vi "Day 3-1.vi"() -> ()   [LabVIEW 2019, in "Day 3.lvlib"]
uses:
  <vilib>/Utility/error.llb/Error Cluster From Error Code.vi
  <vilib>/ErrorRing/Error Ring.xnode
  Day 3.lvlib
panel:
  out "Array 3":bool[][](array[boolean])
  out "x*y":u32
  out "epsilon num":u32
  out "gama num":u32
  out "epsilon":bool[](array[boolean])
  out "gama":bool[](array[boolean])
  out "Array 2":bool[][](array[boolean])
  out "error IO":errorcluster
  out "Array":string[](array[string])
  in  "String":string="010110011101\n101100111000\n100100000011\n111000010001\n001100010011\n010000111100\n001000100011\n001000100111\n010001111110\n111101001011\n011000101011\n111100111001\n100101111011\n101100110110\n101010111001\n001111000110\n001001101000\n101011001010\n011101111010\n011101001010\n011001000001\n100001010000\n111011001101\n000111110111\n010011001111\n000111011001\n111000010100\n101001100100\n110010001101\n111110101000\n011001100010\n110010110101\n010000001101\n100000000100\n110111011110\n110001100110\n001011110111\n110000011110\n110110101010\n101001100110\n010000001010\n100010100100\n101000111101\n111000001011\n000000100100\n100111010110\n01..."
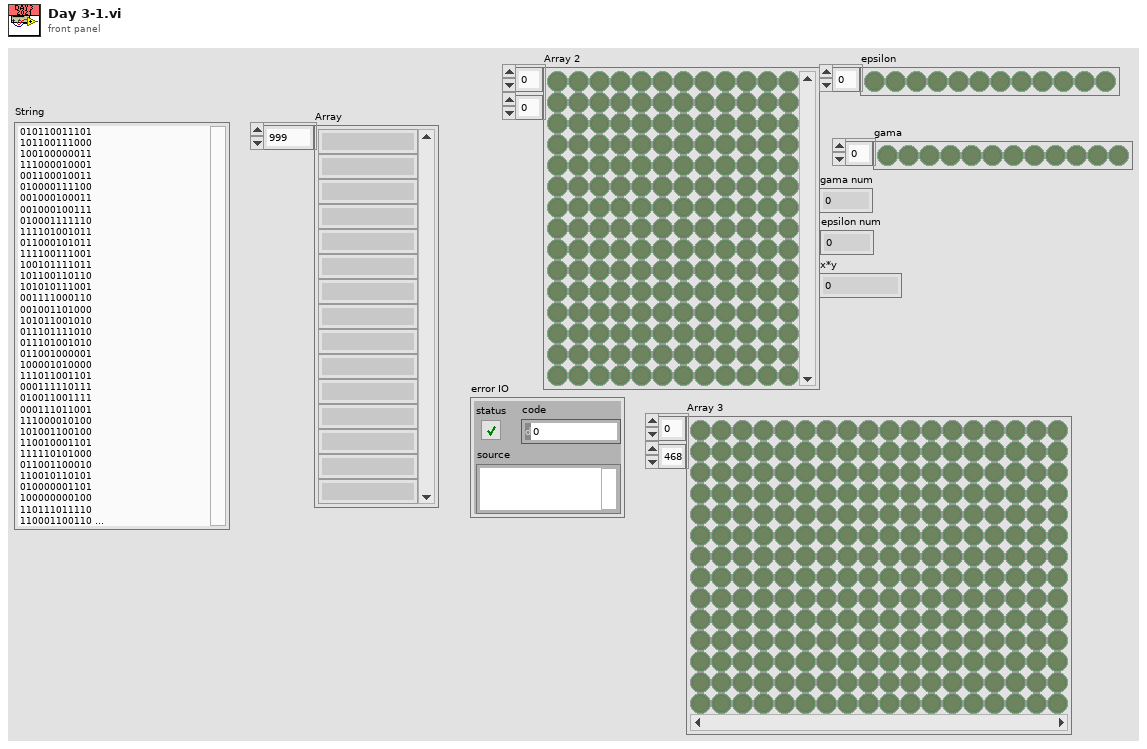
[diagram p1: front panel]
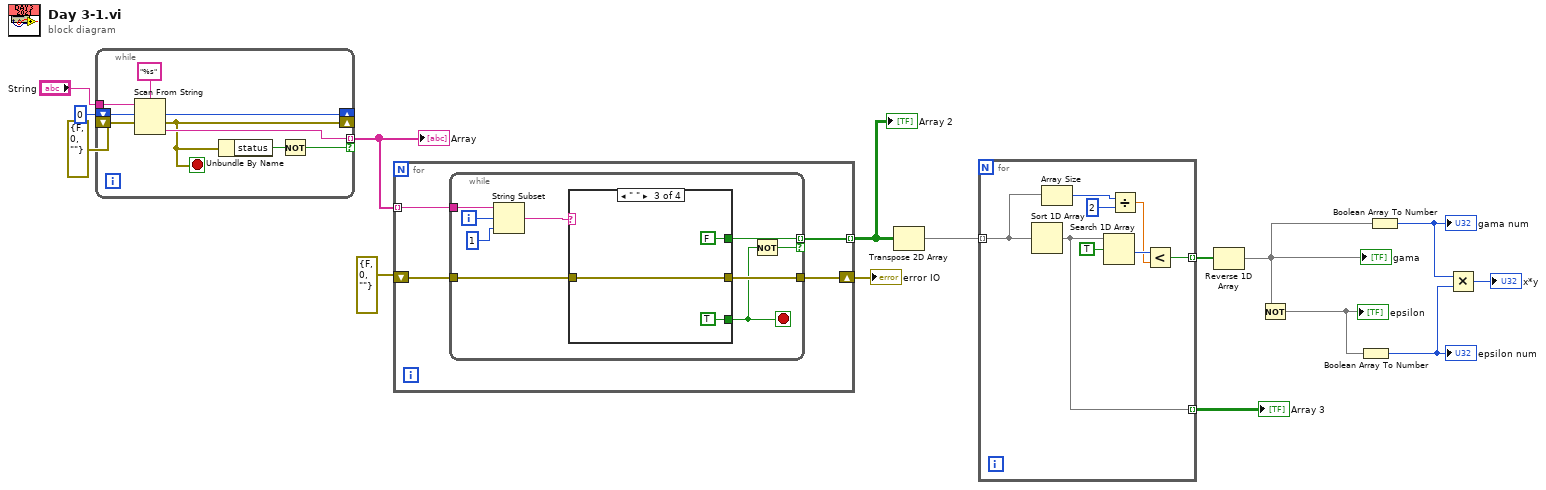
[diagram p0: block diagram]
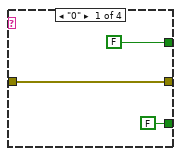
[diagram p2: hidden frame]
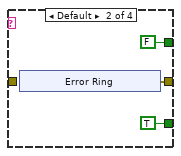
[diagram p3: hidden frame]
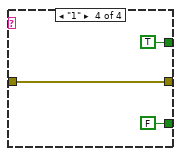
[diagram p4: hidden frame]
diagram:
  n1 = while {
    tunnel: [w22] -> w13 mode=indexing if=w16
    tunnel: "String" -> [w24]
    shift-right: [w19] -> _
    shift-left: u32 0 -> [w21]
    shift-right: [w18] -> _
    shift-left: errorcluster {"status"=FALSE, "code"=0, "source"=""} ("error IO") -> [w20]
    stop <- w18 stop-if-true
    n2 = Scan From String(format string="%s", input string=w24, initial scan location=w21, error in=w20) -> (offset past scan=w19:u32, error out=w18:errorcluster, output 1=w22:string)  [unwired: 1 in, 1 out]
    n3 = Unbundle By Name(w18) -> ("status"=w17:bool)
    n4 = Not(x=w17) -> (.not. x?=w16:bool)
  }
  "Array" <- w13
  n5 = for {
    tunnel: w13 -> [w28] mode=indexing
    shift-right: [w25] -> w12
    shift-left: errorcluster {"status"=FALSE, "code"=0, "source"=""} ("error out") -> [w27]
    tunnel: [w26] -> w9 mode=indexing
    n6 = while {
      tunnel: w28 -> [w37]
      tunnel: w27 -> [w33]
      tunnel: [w32] -> w26 mode=indexing if=w30
      tunnel: [w31] -> w25
      i -> [w36]
      stop <- w29 stop-if-true
      n7 = String Subset(string=w37, offset (0)=w36, length (rest)=1 ("length (rest)")) -> (substring=w34:string)
      n8 = case shown="\" \"" w34 {
        tunnel: [w40 w43 w51 w54] -> w31
        tunnel: w33 -> [w40 _ w51 w54]
        tunnel: [FALSE FALSE FALSE TRUE] -> w32
        tunnel: [FALSE TRUE TRUE FALSE] -> w29
        frame "0" {
        }
        frame Default {
          n9 = xnode "Error Ring"() -> ("error out"=w43:errorcluster)
        }
        frame " " {
        }
        frame "1" {
        }
      }
      n10 = Not(x=w29) -> (.not. x?=w30:bool)
    }
  }
  "error IO" <- w12
  "Array 2" <- w9
  n11 = Transpose 2D Array(2D array=w9) -> (transposed array=w8:bool[][])
  n12 = for {
    tunnel: w8 -> [w61] mode=indexing
    tunnel: [w56] -> w2 mode=indexing
    tunnel: [w55] -> w3 mode=indexing
    n13 = Sort 1D Array(array=w61) -> (sorted array=w55:bool[])
    n14 = Array Size(array=w61) -> (size(s)=w60:i32)
    n15 = Search 1D Array(1D array=w55, element=TRUE) -> (index of element=w58:i32)  [unwired: 1 in]
    n16 = Divide(x=w60, y=2) -> (x/y=w57:dbl)
    n17 = Less?(x=w58, y=w57) -> (x < y?=w56:bool)
  }
  "Array 3" <- w3
  n18 = Reverse 1D Array(array=w2) -> (reversed array=w1:bool[])
  "gama" <- w1
  n19 = Not(x=w1) -> (.not. x?=w7:bool[])
  "epsilon" <- w7
  n20 = Boolean Array To Number(Boolean array=w7) -> (number=w5:u32)
  "epsilon num" <- w5
  n21 = Boolean Array To Number(Boolean array=w1) -> (number=w6:u32)
  "gama num" <- w6
  n22 = Multiply(x=w6, y=w5) -> (x*y=→"x*y":u32)
